vi "Write Open_.vi"(8 "error in (no error)":errorcluster, 10 "Open?":bool, 11 "Set O2 Valve STEP in":refnum<class "Denuder STEP.lvclass">) -> (0 "error out":errorcluster, 3 "Set O2 Valve STEP out":refnum<class "Denuder STEP.lvclass">)   [LabVIEW 2014, in "Denuder STEP.lvclass"]
uses:
  Denuder STEP.lvclass
  Denuder STEP.lvclass/Denuder STEP.ctl
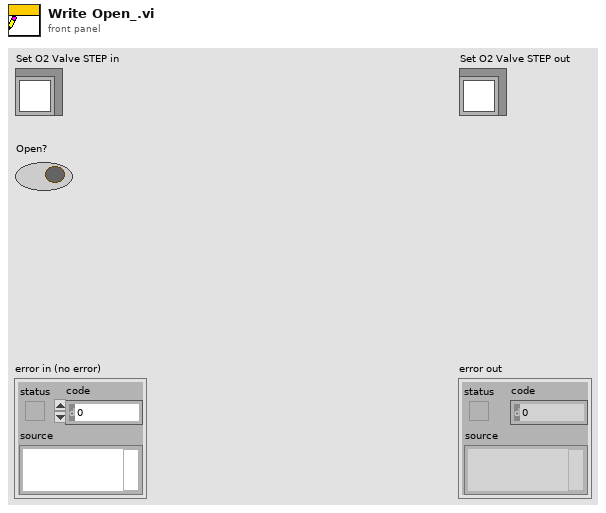
[diagram p1: front panel]
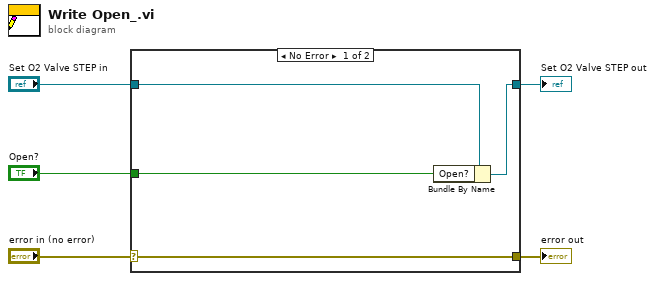
[diagram p0: block diagram]
diagram:
  n1 = case shown="No Error" "error in (no error)" {
    selector: "error in (no error)" -> [w9 w10]
    tunnel: [w9 w10] -> w4
    tunnel: [w7 w11] -> w2
    tunnel: "Set O2 Valve STEP in" -> [w8 w11]
    tunnel: "Open?" -> [w6 _]
    frame No Error {
      n2 = Bundle By Name(cluster=w8, "Open?"=w6) -> (w7:refnum<class "Denuder STEP.lvclass">)
    }
    frame Error {
    }
  }
  "error out" <- w4
  "Set O2 Valve STEP out" <- w2
